vi "gotoOri.vi"(2 "error in":errorcluster, 3 "UART port in":refnum<visa-resource-name>) -> (0 "error out":errorcluster, 1 "UART port out":refnum<visa-resource-name>)   [LabVIEW 2016]
panel:
  out "String 3":string
  out "String 2":string
  out "String":string
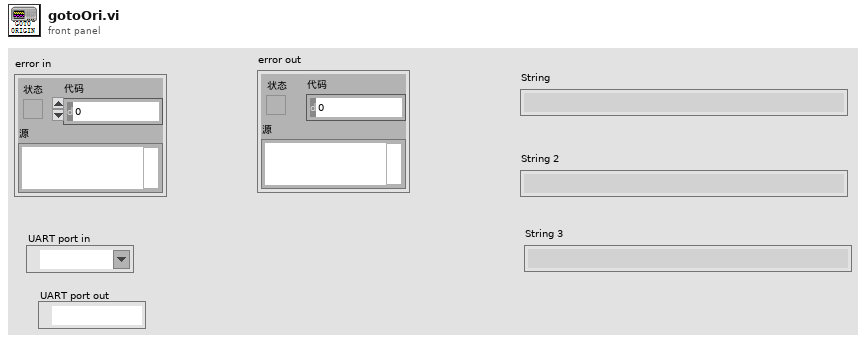
[diagram p1: front panel]
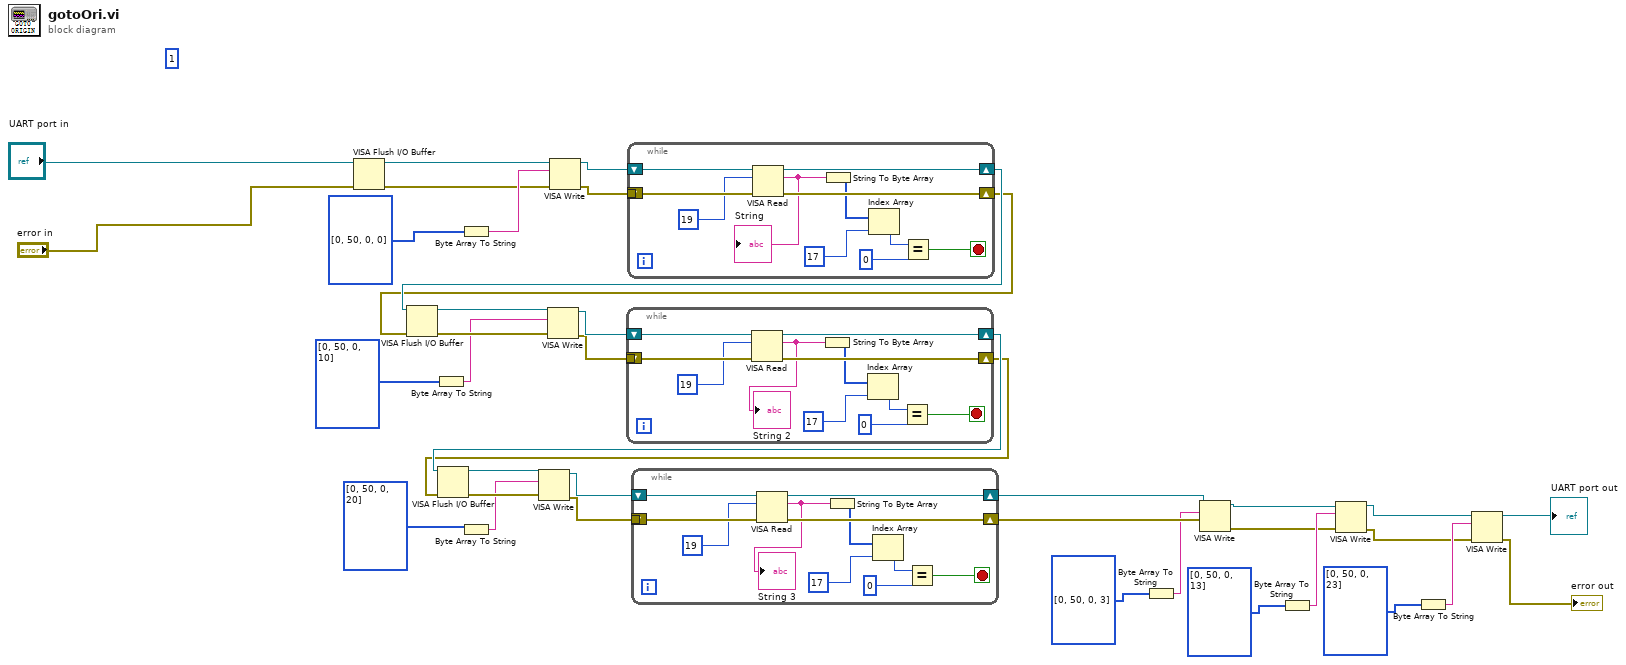
[diagram p0: block diagram]
diagram:
  (unwired) 1
  n1 = VISA Flush I/O Buffer(VISA resource name="UART port in", error in (no error)="error in") -> (VISA resource name out=w36:refnum<visa-resource-name>, error out=w37:errorcluster)  [unwired: 1 in]
  n2 = Byte Array To String(unsigned byte array=i32[] [0, 50, 0, 10]) -> (string=w27:string)
  n3 = Byte Array To String(unsigned byte array=i32[] [0, 50, 0, 0]) -> (string=w38:string)
  n4 = Byte Array To String(unsigned byte array=i32[] [0, 50, 0, 20]) -> (string=w19:string)
  n5 = VISA Write(VISA resource name=w36, write buffer=w38, error in (no error)=w37) -> (VISA resource name out=w34:refnum<visa-resource-name>, error out=w33:errorcluster)  [unwired: 1 out]
  n6 = while {
    tunnel: w33 -> [w48]
    shift-right: [w46] -> w32
    shift-left: w34 -> [w49]
    shift-right: [w45] -> w31
    shift-left: _ -> [_]
    stop <- w42 stop-if-true
    n7 = VISA Read(VISA resource name=w49, byte count=19, error in (no error)=w48) -> (VISA resource name out=w46:refnum<visa-resource-name>, read buffer=w39:string, error out=w45:errorcluster)  [unwired: 1 out]
    "String" <- w39
    n8 = String To Byte Array(string=w39) -> (unsigned byte array=w44:u8[])
    n9 = Index Array(array=w44, index=17) -> (element=w41:u8)
    n10 = Equal?(x=w41, y=0) -> (x = y?=w42:bool)
  }
  n11 = VISA Flush I/O Buffer(VISA resource name=w32, error in (no error)=w31) -> (VISA resource name out=w30:refnum<visa-resource-name>, error out=w29:errorcluster)  [unwired: 1 in]
  n12 = VISA Write(VISA resource name=w30, write buffer=w27, error in (no error)=w29) -> (VISA resource name out=w26:refnum<visa-resource-name>, error out=w25:errorcluster)  [unwired: 1 out]
  n13 = while {
    tunnel: w25 -> [w59]
    shift-right: [w57] -> w24
    shift-left: w26 -> [w60]
    shift-right: [w56] -> w23
    shift-left: _ -> [_]
    stop <- w53 stop-if-true
    n14 = VISA Read(VISA resource name=w60, byte count=19, error in (no error)=w59) -> (VISA resource name out=w57:refnum<visa-resource-name>, read buffer=w50:string, error out=w56:errorcluster)  [unwired: 1 out]
    "String 2" <- w50
    n15 = String To Byte Array(string=w50) -> (unsigned byte array=w55:u8[])
    n16 = Index Array(array=w55, index=17) -> (element=w52:u8)
    n17 = Equal?(x=w52, y=0) -> (x = y?=w53:bool)
  }
  n18 = VISA Flush I/O Buffer(VISA resource name=w24, error in (no error)=w23) -> (VISA resource name out=w21:refnum<visa-resource-name>, error out=w20:errorcluster)  [unwired: 1 in]
  n19 = VISA Write(VISA resource name=w21, write buffer=w19, error in (no error)=w20) -> (VISA resource name out=w18:refnum<visa-resource-name>, error out=w17:errorcluster)  [unwired: 1 out]
  n20 = while {
    tunnel: w17 -> [w70]
    shift-right: [w68] -> w14
    shift-left: w18 -> [w71]
    shift-right: [w67] -> w13
    shift-left: _ -> [_]
    stop <- w64 stop-if-true
    n21 = VISA Read(VISA resource name=w71, byte count=19, error in (no error)=w70) -> (VISA resource name out=w68:refnum<visa-resource-name>, read buffer=w61:string, error out=w67:errorcluster)  [unwired: 1 out]
    "String 3" <- w61
    n22 = String To Byte Array(string=w61) -> (unsigned byte array=w66:u8[])
    n23 = Index Array(array=w66, index=17) -> (element=w63:u8)
    n24 = Equal?(x=w63, y=0) -> (x = y?=w64:bool)
  }
  n25 = Byte Array To String(unsigned byte array=i32[] [0, 50, 0, 3]) -> (string=w11:string)
  n26 = VISA Write(VISA resource name=w14, write buffer=w11, error in (no error)=w13) -> (VISA resource name out=w8:refnum<visa-resource-name>, error out=w7:errorcluster)  [unwired: 1 out]
  n27 = Byte Array To String(unsigned byte array=i32[] [0, 50, 0, 13]) -> (string=w9:string)
  n28 = VISA Write(VISA resource name=w8, write buffer=w9, error in (no error)=w7) -> (VISA resource name out=w3:refnum<visa-resource-name>, error out=w4:errorcluster)  [unwired: 1 out]
  n29 = Byte Array To String(unsigned byte array=i32[] [0, 50, 0, 23]) -> (string=w5:string)
  n30 = VISA Write(VISA resource name=w3, write buffer=w5, error in (no error)=w4) -> (VISA resource name out=→"UART port out":refnum<visa-resource-name>, error out=→"error out":errorcluster)  [unwired: 1 out]
